vi "image_upload.vi"(5 "Extra metadata array":T1(array[cluster])=[{"Attribute"="", "Value"="", "Data type"=enum."<null>"}], 6 "Notes":string, 7 "Tags":string, 8 "Ctl Refnum":refnum<vi>, 10 "Name":string, 11 "Parent ID":string="name") -> (0 "error out":errorcluster, 1 "Saved":bool, 2 "body":string, 3 "headers":string)   [LabVIEW 2013]
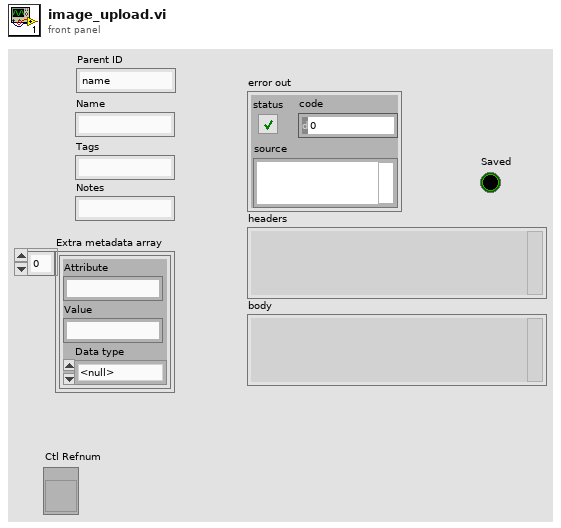
[diagram p1: front panel]
types:
  T1 = cluster{"Attribute":string, "Value":string, "Data type":enum16{"Numeric", "String", "1D array of strings", "1D array of doubles", "Data JSON string", "<null>"}}[]
  T2 = typedef "imagedata.ctl" = cluster{"image type":i32, "image depth":i32, "image":u8[], "mask":u8[], "colors":u32[], "Rectangle":cluster{"left":i16, "top":i16, "right":i16, "bottom":i16}}
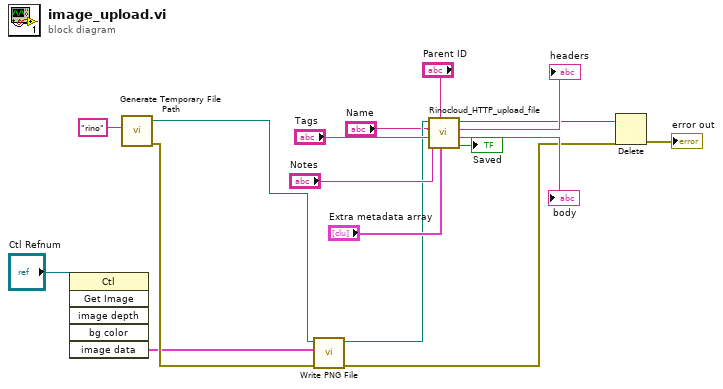
[diagram p0: block diagram]
diagram:
  n1 = invoke class="Ctl" method="Get Image"(reference="Ctl Refnum") -> ("image data"=w3:T2)  [unwired: 5 in, 5 out]
  n2 = call <vilib>:"Generate Temporary File Path.vi"("Temporary File Extension (tmp)"="rino" ("name or relative path")) -> ("error out"=w6:errorcluster, "Unique Temporary File Path"=w8:path)  [unwired: 9 in]
  n3 = call <vilib>:"Write PNG File.vi"("error in (no error)"=w6, "image data"=w3, "path to PNG file"=w8) -> ("error out"=w5:errorcluster, "path"=w7:path)  [unwired: 7 in]
  n4 = call "Rinocloud_HTTP_upload_file.vi"("Extra metadata array"="Extra metadata array", "Parent ID"="Parent ID", "Notes"="Notes", "Tags"="Tags", "Name"="Name", "Path"=w7) -> ("Saved"=→"Saved":bool, "body"=→"body":string, "headers"=→"headers":string, "Path out"=w12:path)  [unwired: 1 in, 1 out]
  n5 = Delete(path (use dialog)=w12, error in=w5) -> (error out=→"error out":errorcluster)  [unwired: 3 in, 2 out]
